vi "Calibrate Power.vi"(9 "quit":bool) -> (0 "Remaining\nMinutes":dbl format="%#.2f", 1 "Finished":bool, 2 "Acquiring":bool, 3 "Waiting":bool, 4 "Current mW":dbl format="%#.0f", 5 "Moving":bool)   [LabVIEW 2010]
uses:
  <vilib>/DAQmx/write.llb/DAQmx Write (Analog Wfm 1Chan NSamp).vi
  <vilib>/DAQmx/write.llb/DAQmx Write (Digital 1D Bool 1Chan 1Samp).vi
  <vilib>/DAQmx/read.llb/DAQmx Read (Analog Wfm 1Chan NSamp).vi
  <vilib>/Utility/file.llb/Write To Spreadsheet File (DBL).vi
  <vilib>/daqmx/miscellaneous.llb/DAQmx Fill In Error Info.vi
  <vilib>/Analysis/NI_AALBase.lvlib
panel:
  out "Scaner":string
  in  "Tab Control":T1(tab)
  out "Min Position":dbl
  out "Max Position":dbl
  out "Current Possition":dbl
  out "Current WV":dbl
  out "?":cluster{i32[], i32[]}(graph)
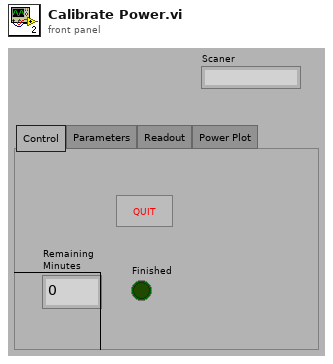
[diagram p1: front panel]
types:
  T1 = enum32{"Control", "Parameters", "Readout", "Power Plot"}
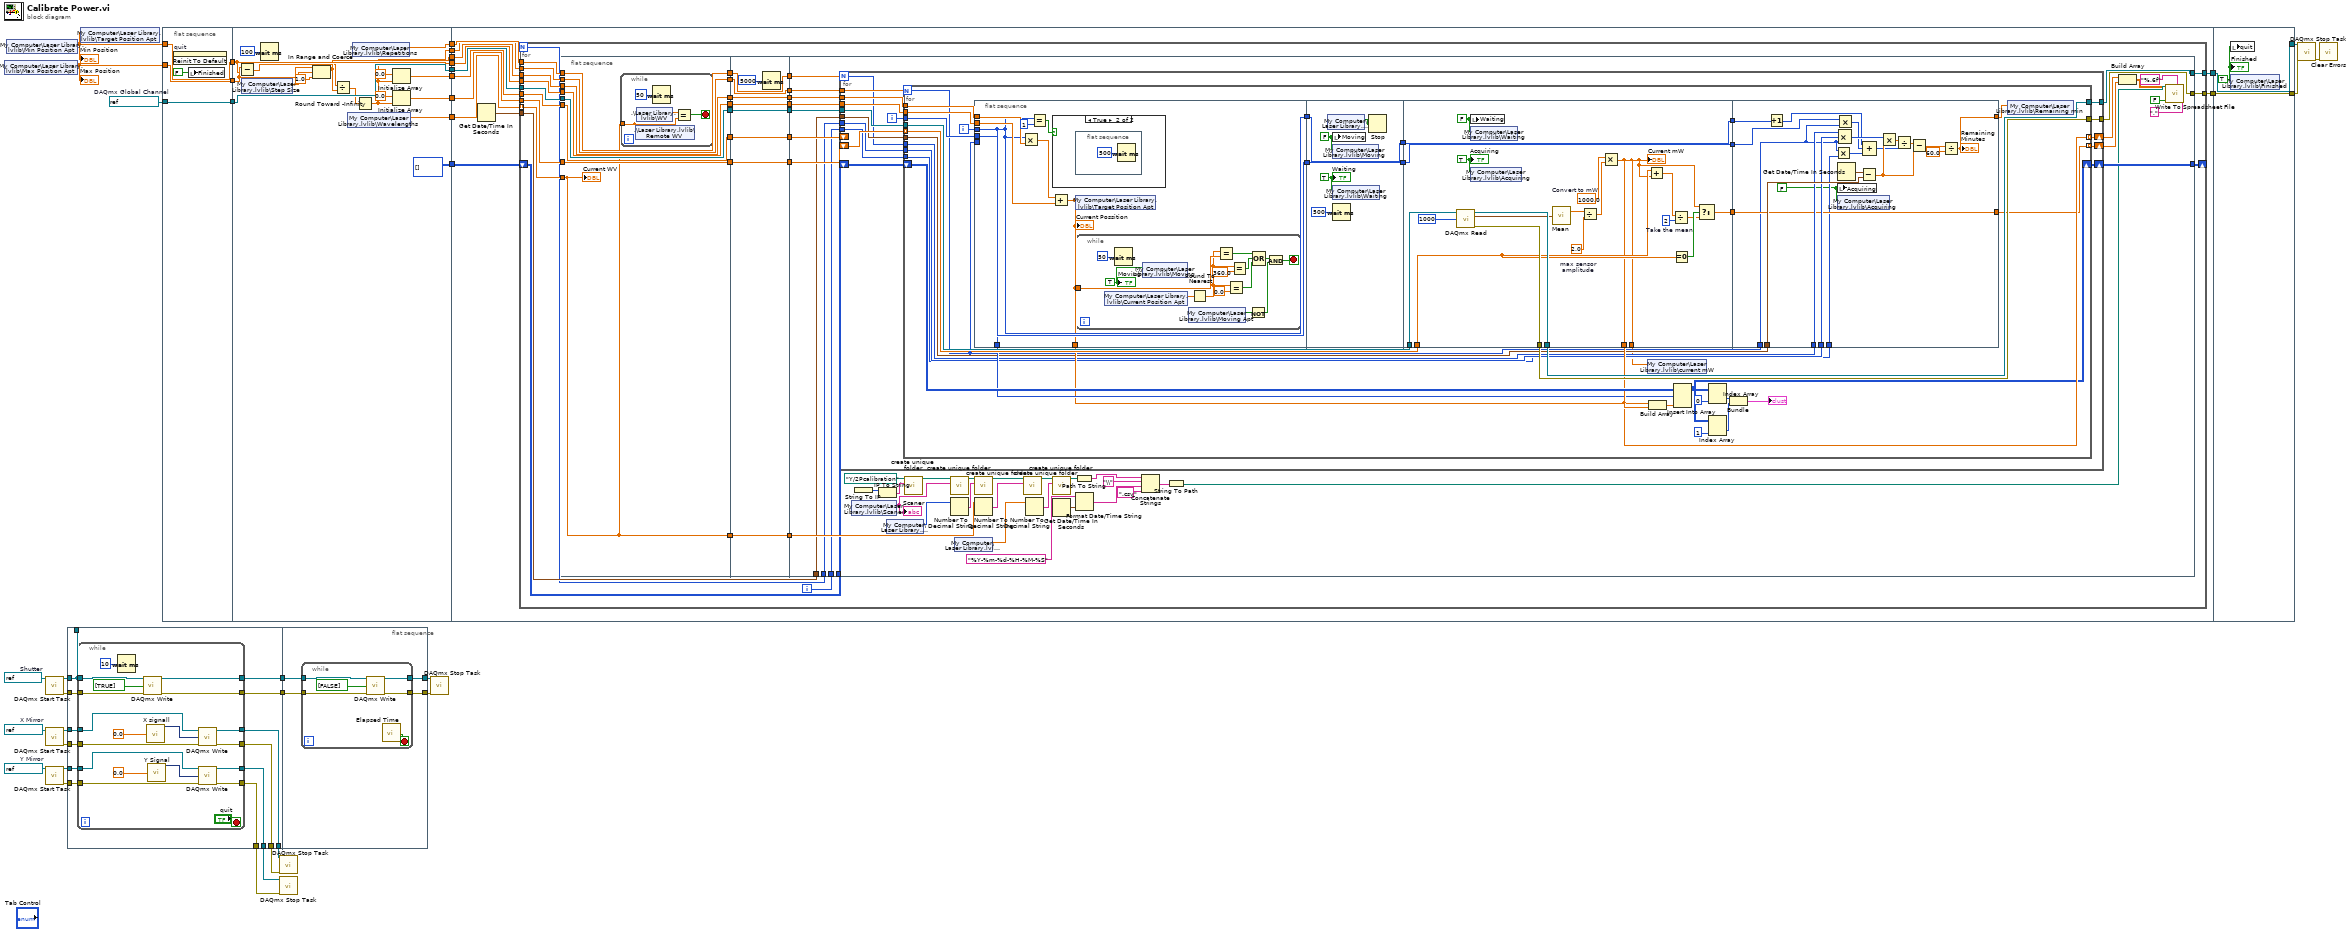
[diagram p0: block diagram]
diagram:
  w11 = refnum<k21> "Y Mirror"  # Y Mirror
  w12 = refnum<k21> "X Mirror"  # X Mirror
  w13 = refnum<k21> "Shutter"  # Shutter
  w20 = refnum<k21> "PowerMeter"  # DAQmx Global Channel
  n1 = shared-variable "My Computer\\Laser Library.lvlib\\Max Position Apt"() -> (w9:dbl)  [unwired: 1 in, 1 out]
  "Max Position" <- w9
  n2 = shared-variable "My Computer\\Laser Library.lvlib\\Min Position Apt"() -> (w10:dbl)  [unwired: 1 in, 1 out]
  "Min Position" <- w10
  n3 = call <vilib>:"DAQmx Start Task.vi"("task/channels in"=w13) -> ("task out"=w5:refnum<k21>, "error out"=w3:errorcluster)  [unwired: 13 in]
  n4 = call <vilib>:"DAQmx Start Task.vi"("task/channels in"=w12) -> ("task out"=w4:refnum<k21>, "error out"=w2:errorcluster)  [unwired: 13 in]
  n5 = call <vilib>:"DAQmx Start Task.vi"("task/channels in"=w11) -> ("task out"=w6:refnum<k21>, "error out"=w1:errorcluster)  [unwired: 13 in]
  n6 = flat-sequence {
    tunnel: [w41] -> _
    tunnel: w4 -> [w49]
    tunnel: [w48] -> w8
    tunnel: [w47] -> w7
    tunnel: [w46] -> w17
    tunnel: [w45] -> w16
    tunnel: [w44] -> w15
    tunnel: [w43] -> w14
    tunnel: w6 -> [w42]
    tunnel: w5 -> [w41]
    tunnel: w3 -> [w40]
    tunnel: w2 -> [w39]
    tunnel: w1 -> [w38]
    tunnel: w8 -> [w72]
    tunnel: [w71] -> w19
    tunnel: [w70] -> w18
    tunnel: w7 -> [w69]
    frame #0 {
      n7 = while {
        tunnel: w41 -> [w62]
        tunnel: w49 -> [w64]
        tunnel: w42 -> [w63]
        tunnel: [w60] -> w48
        tunnel: [w59] -> w47
        tunnel: [w56] -> w46
        tunnel: [w55] -> w45
        tunnel: [w54] -> w44
        tunnel: [w53] -> w43
        tunnel: w40 -> [w52]
        tunnel: w39 -> [w51]
        tunnel: w38 -> [w50]
        stop <- "quit" stop-if-true
        n8 = Wait (ms)(milliseconds to wait=u32 10) -> ()  [unwired: 1 out]
        n9 = call-poly <vilib>:"DAQmx Write.vi"("task/channels in"=w62, "data"=bool[] [TRUE], "error in"=w52) -> ("task out"=w60:refnum<k21>, "error out"=w59:errorcluster)  [unwired: 10 in, 1 out]
        n10 = call "X signall"("Amplitude"=0.0) -> ("Sine"=w58:dynamicdata)  [unwired: 13 in, 1 out]
        n11 = call "Y Signal"("Amplitude"=0.0) -> ("Sine"=w57:dynamicdata)  [unwired: 13 in, 1 out]
        n12 = call-poly <vilib>:"DAQmx Write.vi"("task/channels in"=w64, "data"=w58, "error in"=w51) -> ("task out"=w56:refnum<k21>, "error out"=w55:errorcluster)  [unwired: 10 in, 1 out]
        n13 = call-poly <vilib>:"DAQmx Write.vi"("task/channels in"=w63, "data"=w57, "error in"=w50) -> ("task out"=w54:refnum<k21>, "error out"=w53:errorcluster)  [unwired: 10 in, 1 out]
      }
    }
    frame #1 {
      n14 = while {
        tunnel: w72 -> [w77]
        tunnel: [w75] -> w71
        tunnel: [w74] -> w70
        tunnel: w69 -> [w73]
        stop <- w78 stop-if-true
        n15 = call-poly <vilib>:"DAQmx Write.vi"("task/channels in"=w77, "data"=bool[] [FALSE], "error in"=w73) -> ("task out"=w75:refnum<k21>, "error out"=w74:errorcluster)  [unwired: 10 in, 1 out]
        n16 = call "Elapsed Time"() -> ("Time has Elapsed"=w78:bool)  [unwired: 12 in, 7 out]
      }
    }
  }
  n17 = shared-variable "My Computer\\Laser Library.lvlib\\Target Position Apt"(w10) -> ()  [unwired: 1 in, 1 out]
  n18 = flat-sequence {
    tunnel: w9 -> [w80]
    tunnel: w20 -> [w81]
    tunnel: w10 -> [w82]
    tunnel: [w82] -> w34
    tunnel: [w81] -> w33
    tunnel: [w80] -> w32
    tunnel: [w96] -> w31
    tunnel: [w83] -> w30
    tunnel: [w95] -> w29
    tunnel: [w99] -> w28
    tunnel: [w94] -> w27
    tunnel: [w93] -> w26
    tunnel: [i32[][] []] -> w25
    tunnel: [w85] -> w24
    tunnel: [w92] -> w23
    tunnel: w34 -> [w96]
    tunnel: w33 -> [w99]
    tunnel: w32 -> [w97]
    tunnel: w31 -> [w111]
    tunnel: w30 -> [w110]
    tunnel: w29 -> [w109]
    tunnel: w28 -> [w108]
    tunnel: w27 -> [w106]
    tunnel: w26 -> [w105]
    tunnel: w25 -> [w103]
    tunnel: w24 -> [w104]
    tunnel: w23 -> [w107]
    tunnel: [w102] -> w22
    tunnel: [w101] -> w21
    tunnel: [w328] -> w35
    tunnel: [w329] -> w36
    tunnel: w22 -> [w329]
    tunnel: w21 -> [w328]
    frame #0 {
      n19 = invoke on="quit" class="Bool (strict)" method="Reinit To Default"() -> ()  [unwired: 3 in, 3 out]
      n20 = local write "Finished"(FALSE ("Finished")) -> ()
    }
    frame #1 {
      n21 = Subtract(x=w97, y=w96) -> (x-y=w87:dbl)
      n22 = shared-variable "My Computer\\Laser Library.lvlib\\Step Size"() -> (w84:dbl)  [unwired: 1 in, 1 out]
      n23 = Wait (ms)(milliseconds to wait=u32 100) -> ()  [unwired: 1 out]
      n24 = In Range and Coerce(upper limit=w97, x=w84, lower limit=1.0) -> (coerced(x)=w95:dbl)  [unwired: 1 out]
      n25 = Divide(x=w87, y=w95) -> (x/y=w88:dbl)
      n26 = shared-variable "My Computer\\Laser Library.lvlib\\Wavelengths"() -> (w85:dbl[])  [unwired: 1 in, 1 out]
      n27 = shared-variable "My Computer\\Laser Library.lvlib\\Repetitions"() -> (w83:dbl)  [unwired: 1 in, 1 out]
      n28 = Round Toward -Infinity(1:w88) -> (0:w94:dbl)
      n29 = Initialize Array(0.0 ("element"), w94) -> (w93:dbl[])
      n30 = Initialize Array(0.0 ("element"), w94) -> (w92:dbl[])
    }
    frame #2 {
      n31 = Get Date/Time In Seconds() -> (seconds since 1Jan1904=w100:timestamp)
      n32 = for {
        N -> [w113]
        tunnel: w111 -> [w142]
        tunnel: w110 -> [w141]
        tunnel: w109 -> [w140]
        tunnel: w108 -> [w139]
        tunnel: [w138] -> w102
        tunnel: [w137] -> w101
        tunnel: w107 -> [w136]
        tunnel: w106 -> [w135]
        tunnel: w105 -> [w134]
        tunnel: w104 -> [w133] mode=indexing
        shift-right: [w115] -> _
        shift-left: w103 -> [w116]
        tunnel: w100 -> [w114]
        i -> [w112]
        n33 = flat-sequence {
          tunnel: w133 -> [w143]
          tunnel: w134 -> [w144]
          tunnel: w135 -> [w145]
          tunnel: w136 -> [w146]
          tunnel: w139 -> [w147]
          tunnel: w140 -> [w148]
          tunnel: w141 -> [w149]
          tunnel: w142 -> [w150]
          tunnel: [w150] -> w132
          tunnel: [w149] -> w130
          tunnel: [w148] -> w128
          tunnel: [w147] -> w126
          tunnel: [w146] -> w124
          tunnel: [w145] -> w122
          tunnel: [w144] -> w120
          tunnel: [w143] -> w118
          tunnel: w132 -> [w163]
          tunnel: [w163] -> w131
          tunnel: w130 -> [w162]
          tunnel: [w162] -> w129
          tunnel: w128 -> [w161]
          tunnel: [w161] -> w127
          tunnel: w126 -> [w160]
          tunnel: [w160] -> w125
          tunnel: w124 -> [w159]
          tunnel: [w159] -> w123
          tunnel: w122 -> [w158]
          tunnel: [w158] -> w121
          tunnel: w120 -> [w157]
          tunnel: [w157] -> w119
          tunnel: w118 -> [w156]
          tunnel: [w156] -> w117
          tunnel: [w204] -> w115
          tunnel: [w205] -> w137
          tunnel: [w206] -> w138
          tunnel: w112 -> [w173]
          tunnel: w113 -> [w174]
          tunnel: w114 -> [w175]
          tunnel: w116 -> [w176]
          tunnel: w117 -> [w177]
          tunnel: w119 -> [w197]
          tunnel: w121 -> [w198]
          tunnel: w123 -> [w199]
          tunnel: w125 -> [w200]
          tunnel: w127 -> [w201]
          tunnel: w129 -> [w202]
          tunnel: w131 -> [w203]
          frame #0 {
            n34 = while {
              tunnel: w143 -> [w152]
              stop <- w154 stop-if-true
              n35 = shared-variable ".\\Laser Library.lvlib\\Remote WV"(w152) -> ()  [unwired: 1 in, 1 out]
              n36 = shared-variable ".\\Laser Library.lvlib\\WV"() -> (w151:dbl)  [unwired: 1 in, 1 out]
              n37 = Wait (ms)(milliseconds to wait=u32 50) -> ()  [unwired: 1 out]
              n38 = Equal?(x=w151, y=w152) -> (x = y?=w154:bool)
            }
            "Current WV" <- w143
          }
          frame #1 {
            n39 = Wait (ms)(milliseconds to wait=u32 5000) -> ()  [unwired: 1 out]
          }
          frame #2 {
            n40 = for {
              N: w202 -> [w208]
              tunnel: w198 -> [w222]
              tunnel: w203 -> [w221]
              tunnel: w201 -> [w220]
              tunnel: w200 -> [w219]
              tunnel: [w218] -> w206
              tunnel: [w217] -> w205
              shift-right: [w216] -> w179
              shift-left: w199 -> [w214]
              shift-right: [w215] -> w180
              shift-left: w197 -> [_]
              shift-right: [w213] -> w204
              shift-left: w176 -> [w212]
              tunnel: w175 -> [w210]
              tunnel: w174 -> [w209]
              tunnel: w173 -> [w207]
              i -> [w211]
              n41 = for {
                N: w222 -> [w226]
                tunnel: w221 -> [w256]
                tunnel: w220 -> [w255]
                tunnel: w219 -> [w253]
                tunnel: [w252] -> w218
                tunnel: [w251] -> w217
                tunnel: [w225] -> w216 mode=indexing
                tunnel: w214 -> [w248] mode=indexing
                tunnel: [w244] -> w215 mode=indexing
                shift-right: [w241] -> w213
                shift-left: w212 -> [w249]
                tunnel: w211 -> [w237]
                tunnel: w210 -> [w236]
                tunnel: w209 -> [w235]
                tunnel: w208 -> [w234]
                tunnel: w207 -> [w233]
                i -> [w254]
                n42 = flat-sequence {
                  tunnel: w254 -> [w260]
                  tunnel: w255 -> [w264]
                  tunnel: w256 -> [w261]
                  tunnel: [w257] -> w244
                  tunnel: [w260] -> w245
                  tunnel: w237 -> [w263]
                  tunnel: [w263] -> w230
                  tunnel: [w260] -> w227
                  tunnel: w226 -> [_]
                  tunnel: [w284] -> w231
                  tunnel: w230 -> [w284]
                  tunnel: [w283] -> w228
                  tunnel: w227 -> [w283]
                  tunnel: w253 -> [w305]
                  tunnel: [w304] -> w252
                  tunnel: [w303] -> w251
                  tunnel: w248 -> [w289]
                  tunnel: [w297] -> w250
                  tunnel: [w288] -> w247
                  tunnel: [w291] -> w232
                  tunnel: w231 -> [w291]
                  tunnel: [w290] -> w229
                  tunnel: w228 -> [w290]
                  tunnel: [w288] -> w224
                  tunnel: w250 -> [w320]
                  tunnel: w236 -> [w325]
                  tunnel: w235 -> [w324]
                  tunnel: w234 -> [w323]
                  tunnel: w226 -> [w312]
                  tunnel: w233 -> [w313]
                  tunnel: w232 -> [w314]
                  tunnel: w229 -> [w322]
                  tunnel: [w320] -> w225
                  tunnel: [w307] -> w223
                  frame #0 {
                    n43 = Multiply(x=w260, y=w264) -> (x*y=w262:dbl)
                    n44 = Equal?(x=w260, y=1) -> (x = y?=w259:bool)
                    n45 = case shown="True" w259 {
                      frame False {
                      }
                      frame True {
                        n46 = flat-sequence {
                          frame #0 {
                            n47 = Wait (ms)(milliseconds to wait=u32 500) -> ()  [unwired: 1 out]
                          }
                        }
                      }
                    }
                    n48 = Add(x=w262, y=w261) -> (x+y=w257:dbl)
                    "Current Possition" <- w257
                    n49 = shared-variable "My Computer\\Laser Library.lvlib\\Target Position Apt"(w257) -> ()  [unwired: 1 in, 1 out]
                    n50 = while {
                      tunnel: w257 -> [w278]
                      stop <- w276 stop-if-true
                      w266 = TRUE
                      n51 = shared-variable "My Computer\\Laser Library.lvlib\\Current Position Apt"() -> (w267:dbl)  [unwired: 1 in, 1 out]
                      n52 = Wait (ms)(milliseconds to wait=u32 50) -> ()  [unwired: 1 out]
                      n53 = shared-variable "My Computer\\Laser Library.lvlib\\Moving"(w266) -> ()  [unwired: 1 in, 1 out]
                      n54 = shared-variable "My Computer\\Laser Library.lvlib\\Moving Apt"() -> (w268:bool)  [unwired: 1 in, 1 out]
                      n55 = Round To Nearest(number=w267) -> (nearest integer value=w271:dbl)
                      n56 = Equal?(x=w271, y=w278) -> (x = y?=w275:bool)
                      n57 = Equal?(x=w271, y=0.0) -> (x = y?=w272:bool)
                      n58 = Equal?(x=w271, y=360.0) -> (x = y?=w273:bool)
                      n59 = Not(x=w268) -> (.not. x?=w277:bool)
                      n60 = Compound Arithmetic op=OR(w275, w273, w272) -> (w274:bool)
                      n61 = And(x=w274, y=w277) -> (x .and. y?=w276:bool)
                      "Moving" <- w266
                    }
                  }
                  frame #1 {
                    w281 = TRUE
                    w282 = FALSE
                    n62 = shared-variable "My Computer\\Laser Library.lvlib\\Quit"() -> (w280:bool)  [unwired: 1 in, 1 out]
                    n63 = local write "Moving"(w282) -> ()
                    n64 = shared-variable "My Computer\\Laser Library.lvlib\\Moving"(w282) -> ()  [unwired: 1 in, 1 out]
                    n65 = shared-variable "My Computer\\Laser Library.lvlib\\Waiting"(w281) -> ()  [unwired: 1 in, 1 out]
                    n66 = Wait (ms)(milliseconds to wait=u32 500) -> ()  [unwired: 1 out]
                    n67 = Stop(stop? (T)=w280) -> ()
                    "Waiting" <- w281
                  }
                  frame #2 {
                    w287 = FALSE
                    w292 = 2.0  # max sensor  amplitude
                    w294 = 1000.0  # Convert to mW
                    w300 = 2  # Take the mean
                    w286 = TRUE ("Acquiring")
                    n68 = call-poly <vilib>:"DAQmx Read.vi"("task/channels in"=w305, "number of samples per channel"=1000) -> ("task out"=w304:refnum<k21>, "data"=w295:waveform(dbl), "error out"=w303:errorcluster)  [unwired: 1 in, 10 out]
                    n69 = local write "Waiting"(w287) -> ()
                    n70 = shared-variable "My Computer\\Laser Library.lvlib\\Waiting"(w287) -> ()  [unwired: 1 in, 1 out]
                    n71 = shared-variable "My Computer\\Laser Library.lvlib\\Acquiring"(w286) -> ()  [unwired: 1 in, 1 out]
                    n72 = call <vilib>:"Mean.vi"("X"=w295) -> ("mean"=w296:dbl)  [unwired: 1 out]
                    n73 = Divide(x=w296, y=w292) -> (x/y=w293:dbl)
                    n74 = Multiply(x=w294, y=w293) -> (x*y=w288:dbl)
                    "Current mW" <- w288
                    n75 = Add(x=w289, y=w288) -> (x+y=w299:dbl)
                    n76 = Divide(x=w299, y=w300) -> (x/y=w298:dbl)
                    n77 = Equal To 0?(x=w289) -> (x = 0?=w301:bool)
                    n78 = Select(t=w288, s=w301, f=w298) -> (s? t:f=w297:dbl)
                    "Acquiring" <- w286
                  }
                  frame #3 {
                    w306 = FALSE ("Acquiring")
                    n79 = Increment(x=w322) -> (x+1=w311:i32)
                    n80 = Multiply(x=w312, y=w313) -> (x*y=w309:i32)
                    n81 = Multiply(x=w314, y=w312) -> (x*y=w310:i32)
                    n82 = Get Date/Time In Seconds() -> (seconds since 1Jan1904=w326:timestamp)
                    n83 = local write "Acquiring"(w306) -> ()
                    n84 = shared-variable "My Computer\\Laser Library.lvlib\\Acquiring"(w306) -> ()  [unwired: 1 in, 1 out]
                    n85 = Compound Arithmetic op=MULTIPLY(w323, w324, w312) -> (w319:i32)
                    n86 = Subtract(x=w326, y=w325) -> (x-y=w317:dbl)
                    n87 = Compound Arithmetic op=ADD(w311, w310, w309) -> (w308:i32)
                    n88 = Multiply(x=w319, y=w317) -> (x*y=w318:dbl)
                    n89 = Divide(x=w318, y=w308) -> (x/y=w316:dbl)
                    n90 = Subtract(x=w316, y=w317) -> (x-y=w315:dbl)
                    n91 = Divide(x=w315, y=60.0) -> (x/y=w307:dbl)
                    "Remaining\nMinutes" <- w307
                  }
                }
                n92 = shared-variable "My Computer\\Laser Library.lvlib\\current mW"(w224) -> ()  [unwired: 1 in, 1 out]
                n93 = Build Array(w244, w247) -> (w246:dbl[])
                n94 = Insert Into Array(array=w249, index (row)=w245, new element=w246) -> (w241:i32[][])  [unwired: 1 in]
                n95 = Index Array(array=w241, index (col)=0 ("index")) -> (element=w242:i32[])  [unwired: 1 in]
                n96 = Index Array(array=w241, index (col)=1 ("index")) -> (element=w239:i32[])  [unwired: 1 in]
                n97 = Bundle(w242, w239) -> (→"?":cluster{i32[], i32[]})  [unwired: 1 in]
                n98 = shared-variable "My Computer\\Laser Library.lvlib\\Remaining min"(w223) -> ()  [unwired: 1 in, 1 out]
              }
            }
            n99 = shared-variable "My Computer\\Laser Library.lvlib\\Scaner"() -> (w168:string)  [unwired: 1 in, 1 out]
            "Scaner" <- w168
            n100 = String To IP() -> (0:w190:u32)  [unwired: 1 in]
            n101 = IP To String(2:w190) -> (0:w172:string)  [unwired: 1 in]
            n102 = shared-variable "My Computer\\Laser Library.lvlib\\lens"() -> (w171:u16)  [unwired: 1 in, 1 out]
            n103 = call "create unique folder.vi"("string"=w172, "path 2"=path "Y:/2Pcalibration") -> ("path"=w170:path)  [unwired: 9 in]
            n104 = call "create unique folder.vi"("string"=w168, "path 2"=w170) -> ("path"=w169:path)  [unwired: 9 in]
            n105 = Number To Decimal String(number=w171) -> (decimal integer string=w181:string)  [unwired: 1 in]
            n106 = shared-variable "My Computer\\Laser Library.lvlib\\GDD"() -> (w167:dbl)  [unwired: 1 in, 1 out]
            n107 = call "create unique folder.vi"("string"=w181, "path 2"=w169) -> ("path"=w182:path)  [unwired: 9 in]
            n108 = Number To Decimal String(number=w177) -> (decimal integer string=w189:string)  [unwired: 1 in]
            n109 = call "create unique folder.vi"("string"=w189, "path 2"=w182) -> ("path"=w166:path)  [unwired: 9 in]
            n110 = Number To Decimal String(number=w167) -> (decimal integer string=w164:string)  [unwired: 1 in]
            n111 = call "create unique folder.vi"("string"=w164, "path 2"=w166) -> ("path"=w165:path)  [unwired: 9 in]
            n112 = Get Date/Time In Seconds() -> (seconds since 1Jan1904=w193:timestamp)
            n113 = Path To String(path=w165) -> (string=w188:string)
            n114 = Format Date/Time String(time format string (%c)="%Y-%m-%d-%H-%M-%S", seconds (now)=w193) -> (date/time string=w186:string)  [unwired: 1 in]
            n115 = Concatenate Strings(w188, "\\" ("string"), w186, ".csv" ("string")) -> (w185:string)
            n116 = String To Path(string=w185) -> (path=w184:path)
            n117 = Build Array(w180, w179) -> (w178:dbl[][])
            n118 = call-poly <vilib>:"Write To Spreadsheet File.vi"("delimiter (\\t)"="," ("delimiter (\\t)"), "format (%.3f)"="%.6f", "append to file? (new file:F)"=FALSE, "2D data"=w178, "file path (dialog if empty)"=w184) -> ()  [unwired: 2 in, 2 out]
          }
        }
      }
    }
    frame #3 {
      w327 = TRUE ("Finished")
      n119 = local write "quit"(w327) -> ()
      n120 = shared-variable "My Computer\\Laser Library.lvlib\\Finished"(w327) -> ()  [unwired: 1 in, 1 out]
      "Finished" <- w327
    }
  }
  n121 = call <vilib>:"DAQmx Stop Task.vi"("task/channels in"=w17, "error in"=w16) -> ()  [unwired: 12 in, 2 out]
  n122 = call <vilib>:"DAQmx Stop Task.vi"("task/channels in"=w15, "error in"=w14) -> ()  [unwired: 12 in, 2 out]
  n123 = call <vilib>:"DAQmx Stop Task.vi"("task/channels in"=w19, "error in"=w18) -> ()  [unwired: 12 in, 2 out]
  n124 = call <vilib>:"DAQmx Stop Task.vi"("task/channels in"=w36, "error in"=w35) -> ("error out"=w37:errorcluster)  [unwired: 13 out]
  n125 = call <vilib>:"Clear Errors.vi"("error in (no error)"=w37) -> ()  [unwired: 6 in, 1 out]
